vi "IX83 Test Panel.vi"() -> ()   [LabVIEW 2020]
uses:
  5a02a602-ae61-46a8-970d-d46dffe540ac.vi
panel:
  out "EXE Path":path
  out "FP Reply":string
  out "Connected":bool
  in  "Quit":bool
  in  "Command":string
  out "Reply":string
  out "Value":dbl
  out "Bool":bool
  in  "Wait for Reply":bool=TRUE
  out "Command History":string
  out "Waiting for Reply":bool
  out "Cmd Success":bool
  out "Last Error":errorcluster
  out "Trim Reply":string
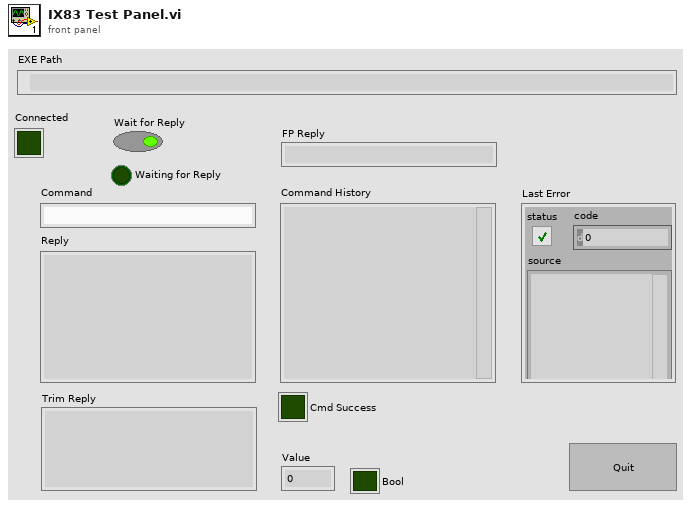
[diagram p1: front panel]
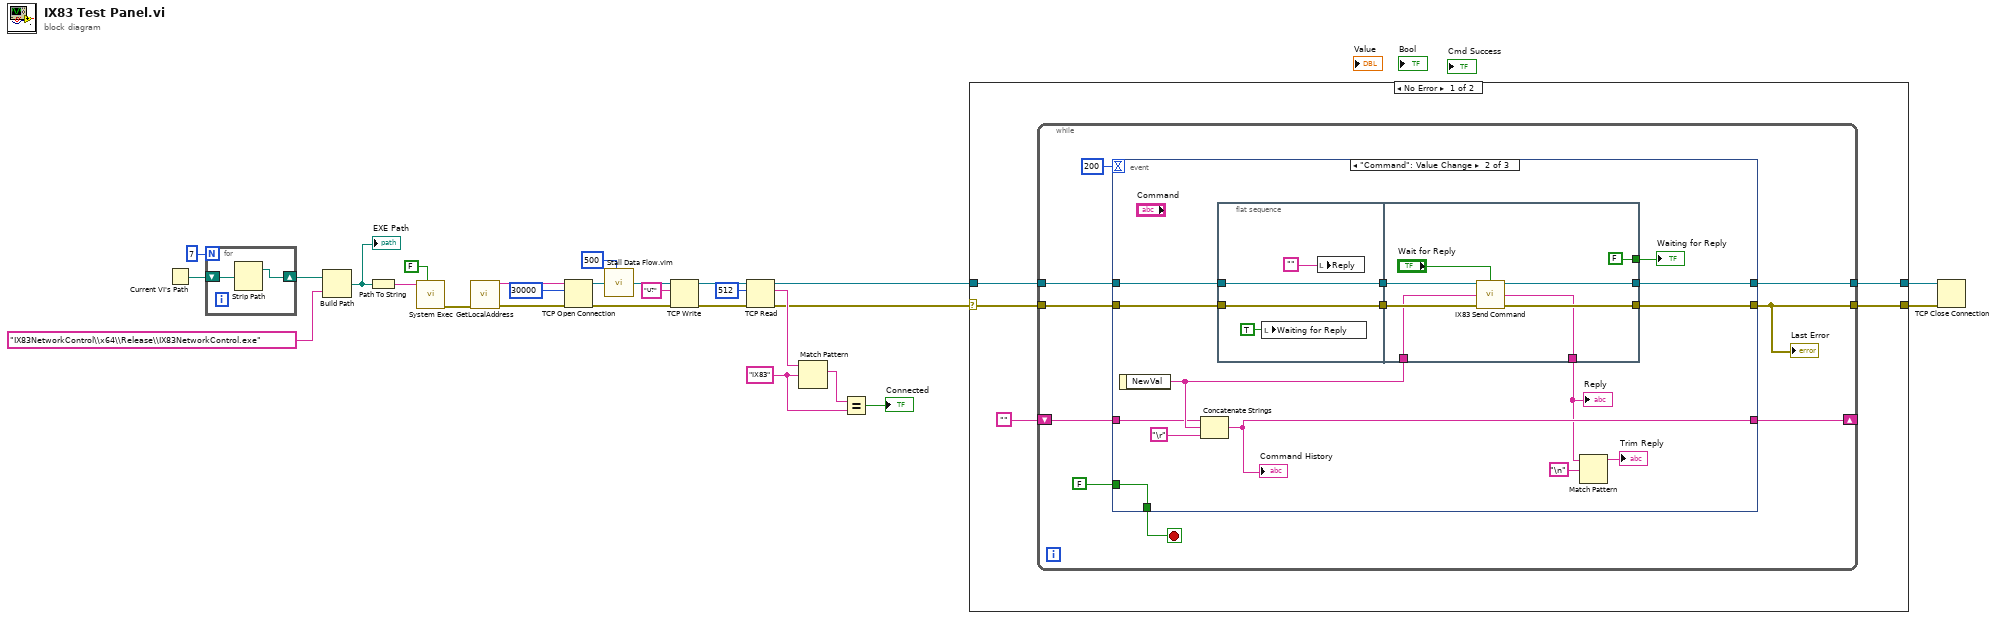
[diagram p0: block diagram]
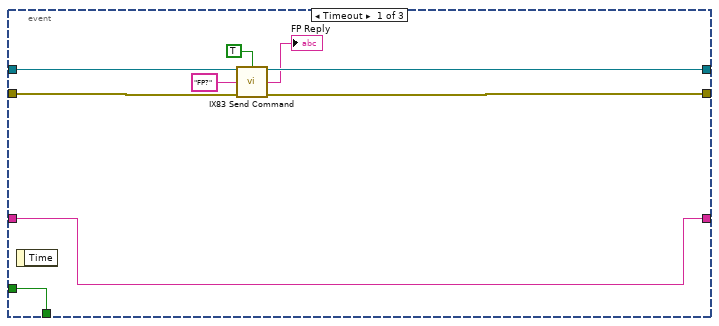
[diagram p2: hidden frame]
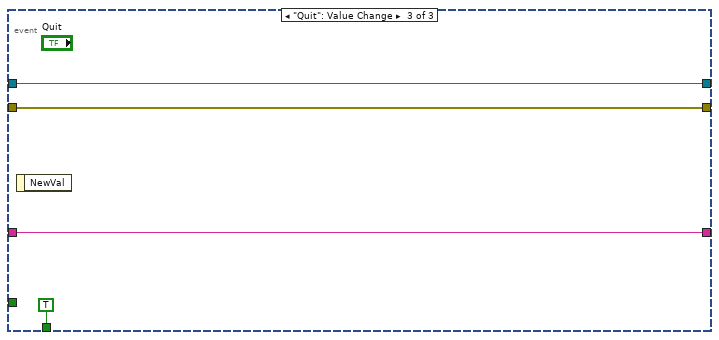
[diagram p3: hidden frame]
diagram:
  w12 = "IX83" ("regular expression")
  n1 = Current VI's Path() -> (path=w5:path)
  n2 = for {
    N: 7 -> [_]
    shift-right: [w28] -> w3
    shift-left: w5 -> [w29]
    n3 = Strip Path(path=w29) -> (stripped path=w28:path)  [unwired: 1 out]
  }
  n4 = Build Path(base path=w3, name or relative path="IX83NetworkControl\\x64\\Release\\IX83NetworkControl.exe") -> (appended path=w1:path)
  "EXE Path" <- w1
  n5 = Path To String(path=w1) -> (string=w26:string)
  n6 = call <vilib>:"System Exec.vi"("wait until completion? (T)"=FALSE, "command line"=w26) -> ("error out"=w24:errorcluster)  [unwired: 6 in, 3 out]
  n7 = call "GetLocalAddress.vi"("Error In"=w24) -> ("IP Address"=w23:string, "Error Out"=w22:errorcluster)  [unwired: 13 in]
  n8 = TCP Open Connection(address=w23, remote port or service name=u16 30000, error in (no error)=w22) -> (connection ID=w7:refnum<k5>, error out=w19:errorcluster)  [unwired: 2 in]
  n9 = call "Stall Data Flow.vim"("value in"=w7, "milliseconds to wait"=u32 500) -> ("value out"=w6:refnum<k5>)  [unwired: 1 out]
  n10 = TCP Write(connection ID=w6, data in="U?", error in (no error)=w19) -> (connection ID out=w15:refnum<k5>, error out=w16:errorcluster)  [unwired: 1 in, 1 out]
  n11 = TCP Read(connection ID=w15, bytes to read=512, error in (no error)=w16) -> (connection ID out=w10:refnum<k5>, data out=w14:string, error out=w9:errorcluster)  [unwired: 2 in]
  n12 = Match Pattern(string=w14, regular expression=w12) -> (match substring=w13:string)  [unwired: 1 in, 3 out]
  n13 = Equal?(x=w13, y=w12) -> (x = y?=→"Connected":bool)
  n14 = case shown="No Error" w9 {
    selector: w9 -> [w33 w84]
    tunnel: w10 -> [w34 w85]
    tunnel: [w32 w85] -> w21
    tunnel: [w31 w84] -> w20
    frame No Error {
      n15 = while {
        tunnel: w34 -> [w41]
        tunnel: w33 -> [w40]
        tunnel: [w39] -> w32
        tunnel: [w36] -> w31
        shift-right: [w37] -> _
        shift-left: "" -> [w38]
        stop <- w42 stop-if-true
        n16 = event shown="[1] \"Command\": Value Change" {
          selector: _ -> [_ _ _]
          dyn-events: _ -> [_ _ _]
          timeout: 200 -> [_ _ _]
          tunnel: FALSE -> [w52 w67 _]
          tunnel: [w52 w67 TRUE] -> w42
          tunnel: w41 -> [w50 w66 w83]
          tunnel: w40 -> [w48 w65 w82]
          tunnel: [w49 w61 w83] -> w39
          tunnel: [w46 w62 w82] -> w36
          tunnel: w38 -> [w51 w58 w80]
          tunnel: [w51 w57 w80] -> w37
          event Timeout {
            n17 = event-data() -> ()  [unwired: 1 in, 1 out]
            n18 = call "IX83 Send Command.vi"("Connection ID"=w50, "Wait for Reply"=TRUE, "Cmd"="FP?" ("data in"), "Error In"=w48) -> ("Connection ID Out"=w49:refnum<k5>, "CMD Reply"=→"FP Reply":string, "Error Out"=w46:errorcluster)  [unwired: 9 in]
          }
          event "Command": Value Change {
            n19 = event-data() -> ("NewVal"=w60:string)  [unwired: 1 in]
            n20 = Concatenate Strings(w58, w60, "\r") -> (w57:string)
            "Command History" <- w57
            n21 = flat-sequence {
              tunnel: w65 -> [w70]
              tunnel: w66 -> [w71]
              tunnel: [w71] -> w64
              tunnel: [w70] -> w63
              tunnel: w60 -> [w73]
              tunnel: w64 -> [w78]
              tunnel: w63 -> [w76]
              tunnel: [w74] -> w62
              tunnel: [w75] -> w61
              tunnel: [FALSE] -> w56
              tunnel: [w72] -> w53
              frame #0 {
                n22 = local write "Waiting for Reply"(TRUE ("Waiting for Cmd")) -> ()
                n23 = local write "Reply"("") -> ()
              }
              frame #1 {
                n24 = call "IX83 Send Command.vi"("Connection ID"=w78, "Wait for Reply"="Wait for Reply", "Cmd"=w73, "Error In"=w76) -> ("Connection ID Out"=w75:refnum<k5>, "CMD Reply"=w72:string, "Error Out"=w74:errorcluster)  [unwired: 9 in]
              }
            }
            n25 = Match Pattern(string=w53, regular expression="\n") -> (before substring=→"Trim Reply":string)  [unwired: 1 in, 3 out]
            "Waiting for Reply" <- w56
            "Reply" <- w53
          }
          event "Quit": Value Change {
            n26 = event-data() -> ()  [unwired: 1 in, 1 out]
          }
        }
        "Last Error" <- w36
      }
    }
    frame Error {
    }
  }
  n27 = TCP Close Connection(connection ID=w21, error in (no error)=w20) -> ()  [unwired: 1 in, 2 out]
